vi "Initialize (Helper).vi"(5 "Password":string, 6 "Connect Timeout (4000 ms)":u32=4000, 7 "User Name":string, 8 "error in (no error)":errorcluster, 9 "Language (Automatic)":T1 items=["Automatic"=0, "Chinese Simplified"=2052, "English"=1033, "French"=1036, "German"=1031, "Japanese"=1041, "Korean"=1042], 10 "Force Property Refresh (T)":bool=TRUE, 11 "Session in":refnum<k21>) -> (0 "error out":errorcluster, 3 "Session out":refnum<k21>)   [LabVIEW 2017, in "nisyscfg.lvlib"]
uses:
  <vilib>/nisyscfg/nisyscfg.lvlib
  <vilib>/nisyscfg/Language.ctl
  <vilib>/Utility/error.llb/Error Cluster From Error Code.vi
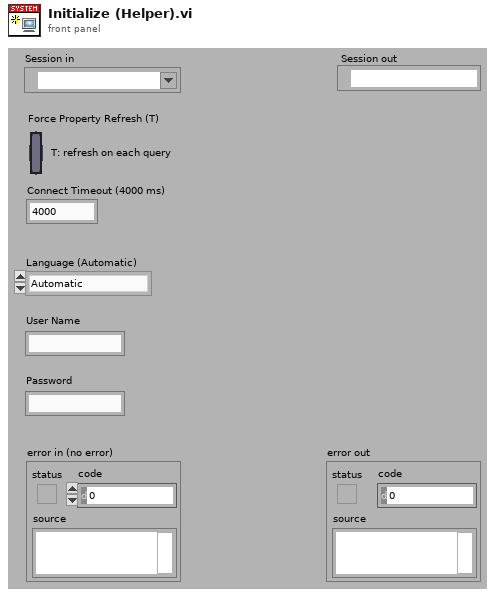
[diagram p1: front panel]
types:
  T1 = typedef "nisyscfg.lvlib/Language.ctl" = i32
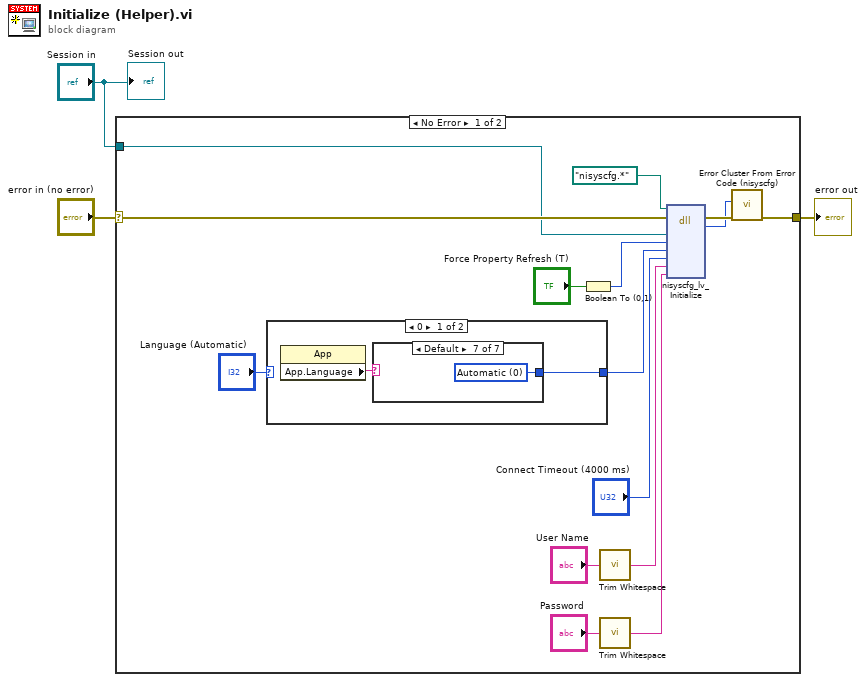
[diagram p0: block diagram]
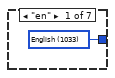
[diagram p2: hidden frame]
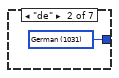
[diagram p3: hidden frame]
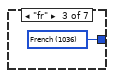
[diagram p4: hidden frame]
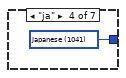
[diagram p5: hidden frame]
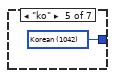
[diagram p6: hidden frame]
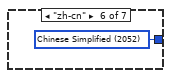
[diagram p7: hidden frame]
diagram:
  n1 = case shown="No Error" "error in (no error)" {
    selector: "error in (no error)" -> [w12 w29]
    tunnel: [w5 w29] -> w3
    tunnel: "Session in" -> [w11 _]
    frame No Error {
      n2 = case shown="0" "Language (Automatic)" {
        selector: "Language (Automatic)" -> [_ w28]
        tunnel: [w19 w28] -> w13
        frame 0 {
          n3 = property class="App"() -> ("App.Language"=w20:string)  [unwired: 2 in, 2 out]
          n4 = case shown="Default" w20 {
            tunnel: [w21 w22 w23 w24 w25 w26 w27] -> w19
            frame "en" {
              w21 = 1033 items=["Automatic"=0, "Chinese Simplified"=2052, "English"=1033, "French"=1036, "German"=1031, "Japanese"=1041, "Korean"=1042] ("language (automatic)")
            }
            frame "de" {
              w22 = 1031 items=["Automatic"=0, "Chinese Simplified"=2052, "English"=1033, "French"=1036, "German"=1031, "Japanese"=1041, "Korean"=1042] ("language (automatic)")
            }
            frame "fr" {
              w23 = 1036 items=["Automatic"=0, "Chinese Simplified"=2052, "English"=1033, "French"=1036, "German"=1031, "Japanese"=1041, "Korean"=1042] ("language (automatic)")
            }
            frame "ja" {
              w24 = 1041 items=["Automatic"=0, "Chinese Simplified"=2052, "English"=1033, "French"=1036, "German"=1031, "Japanese"=1041, "Korean"=1042] ("language (automatic)")
            }
            frame "ko" {
              w25 = 1042 items=["Automatic"=0, "Chinese Simplified"=2052, "English"=1033, "French"=1036, "German"=1031, "Japanese"=1041, "Korean"=1042] ("language (automatic)")
            }
            frame "zh-cn" {
              w26 = 2052 items=["Automatic"=0, "Chinese Simplified"=2052, "English"=1033, "French"=1036, "German"=1031, "Japanese"=1041, "Korean"=1042] ("language (automatic)")
            }
            frame Default {
              w27 = 0 items=["Automatic"=0, "Chinese Simplified"=2052, "English"=1033, "French"=1036, "German"=1031, "Japanese"=1041, "Korean"=1042] ("language (automatic)")
            }
          }
        }
        frame Default {
        }
      }
      n5 = Boolean To (0,1)(Boolean="Force Property Refresh (T)") -> (0, 1=w15:i16)
      n6 = call <vilib>:"Trim Whitespace.vi"("string"="User Name") -> ("trimmed string"=w9:string)  [unwired: 1 in]
      n7 = call <vilib>:"Trim Whitespace.vi"("string"="Password") -> ("trimmed string"=w8:string)  [unwired: 1 in]
      n8 = dll-call lib="nisyscfg.*" fn="nisyscfg_lv_Initialize" label="Initialize"(path in=path "nisyscfg.*", error in=w12, "sessionHandle"=w11, "forcePropertyRefresh"=w15, "language"=w13, "connectTimeoutMsec"="Connect Timeout (4000 ms)", "username"=w9, "password"=w8) -> (error out=w6:errorcluster, "status"=w4:i32)  [unwired: 2 in, 6 out]
      n9 = call <vilib>:"Error Cluster From Error Code (nisyscfg).vi"("error in (no error)"=w6, "Error Code (0)"=w4) -> ("error out"=w5:errorcluster)  [unwired: 9 in]
    }
    frame Error {
    }
  }
  "error out" <- w3
  "Session out" <- "Session in"
